vi "Example FPGA Main.vi"() -> ()   [LabVIEW 2010]
uses:
  <vilib>/Platform/TimedLoop/XDataNode/XDataNode.xnode
  <vilib>/Platform/TimedLoop/XDataNode/timing_clust.ctl
  <vilib>/Platform/TimedLoop/XDataNode/nitl_modes.ctl
  <vilib>/Platform/TimedLoop/XDataNode/wakeup.ctl
  <vilib>/Platform/TimedLoop/XDataNode/XDNodeRunTimeDep.lvlib
  <vilib>/NI Veristand/FPGA/NI_VS FPGA Support.lvlib
  <userlib>/_NI VeriStand FPGA Support/NI VeriStand FPGA Clock Support/NI_VS FPGA Clock Support.lvlib
panel:
  in  "PWM9 In Timeout":u32=40000
  out "PWM9 In DC Packet":u64
  out "PWM9 In Freq Packet":u64
  in  "PWM10 In Timeout":u32=40000
  out "PWM10 In DC Packet":u64
  out "PWM10 In Freq Packet":u64
  in  "PWM11 In Timeout":u32=40000
  out "PWM11 In DC Packet":u64
  out "PWM11 In Freq Packet":u64
  in  "PWM8 In Timeout":u32=40000
  out "PWM8 In DC Packet":u64
  out "PWM8 In Freq Packet":u64
  in  "PWM7 In Timeout":u32=40000
  out "PWM7 In DC Packet":u64
  out "PWM7 In Freq Packet":u64
  out "PWM6 In Freq Packet":u64
  in  "PWM6 In Timeout":u32=40000
  out "PWM6 In DC Packet":u64
  in  "Freq_Variable Freq Pkt":u64
  in  "DC Param DO5":u32
  in  "DC Param DO4":u32
  in  "Freq Param DO2":u32
  in  "Freq Param DO3":u32
  in  "DC_Variable DC Pkt":u64
  in  "Both_Variable DC Pkt":u64
  in  "Both_Variable Freq Pkt":u64
  in  "Generate IRQ":bool
  in  "Use External Timing":bool
  in  "Write to  RTSI":bool
  in  "Loop Rate (usec)":u32
  in  "Start":bool
  # "Pulse Generation"
  # "Pulse Generation"
  # "Configuration"
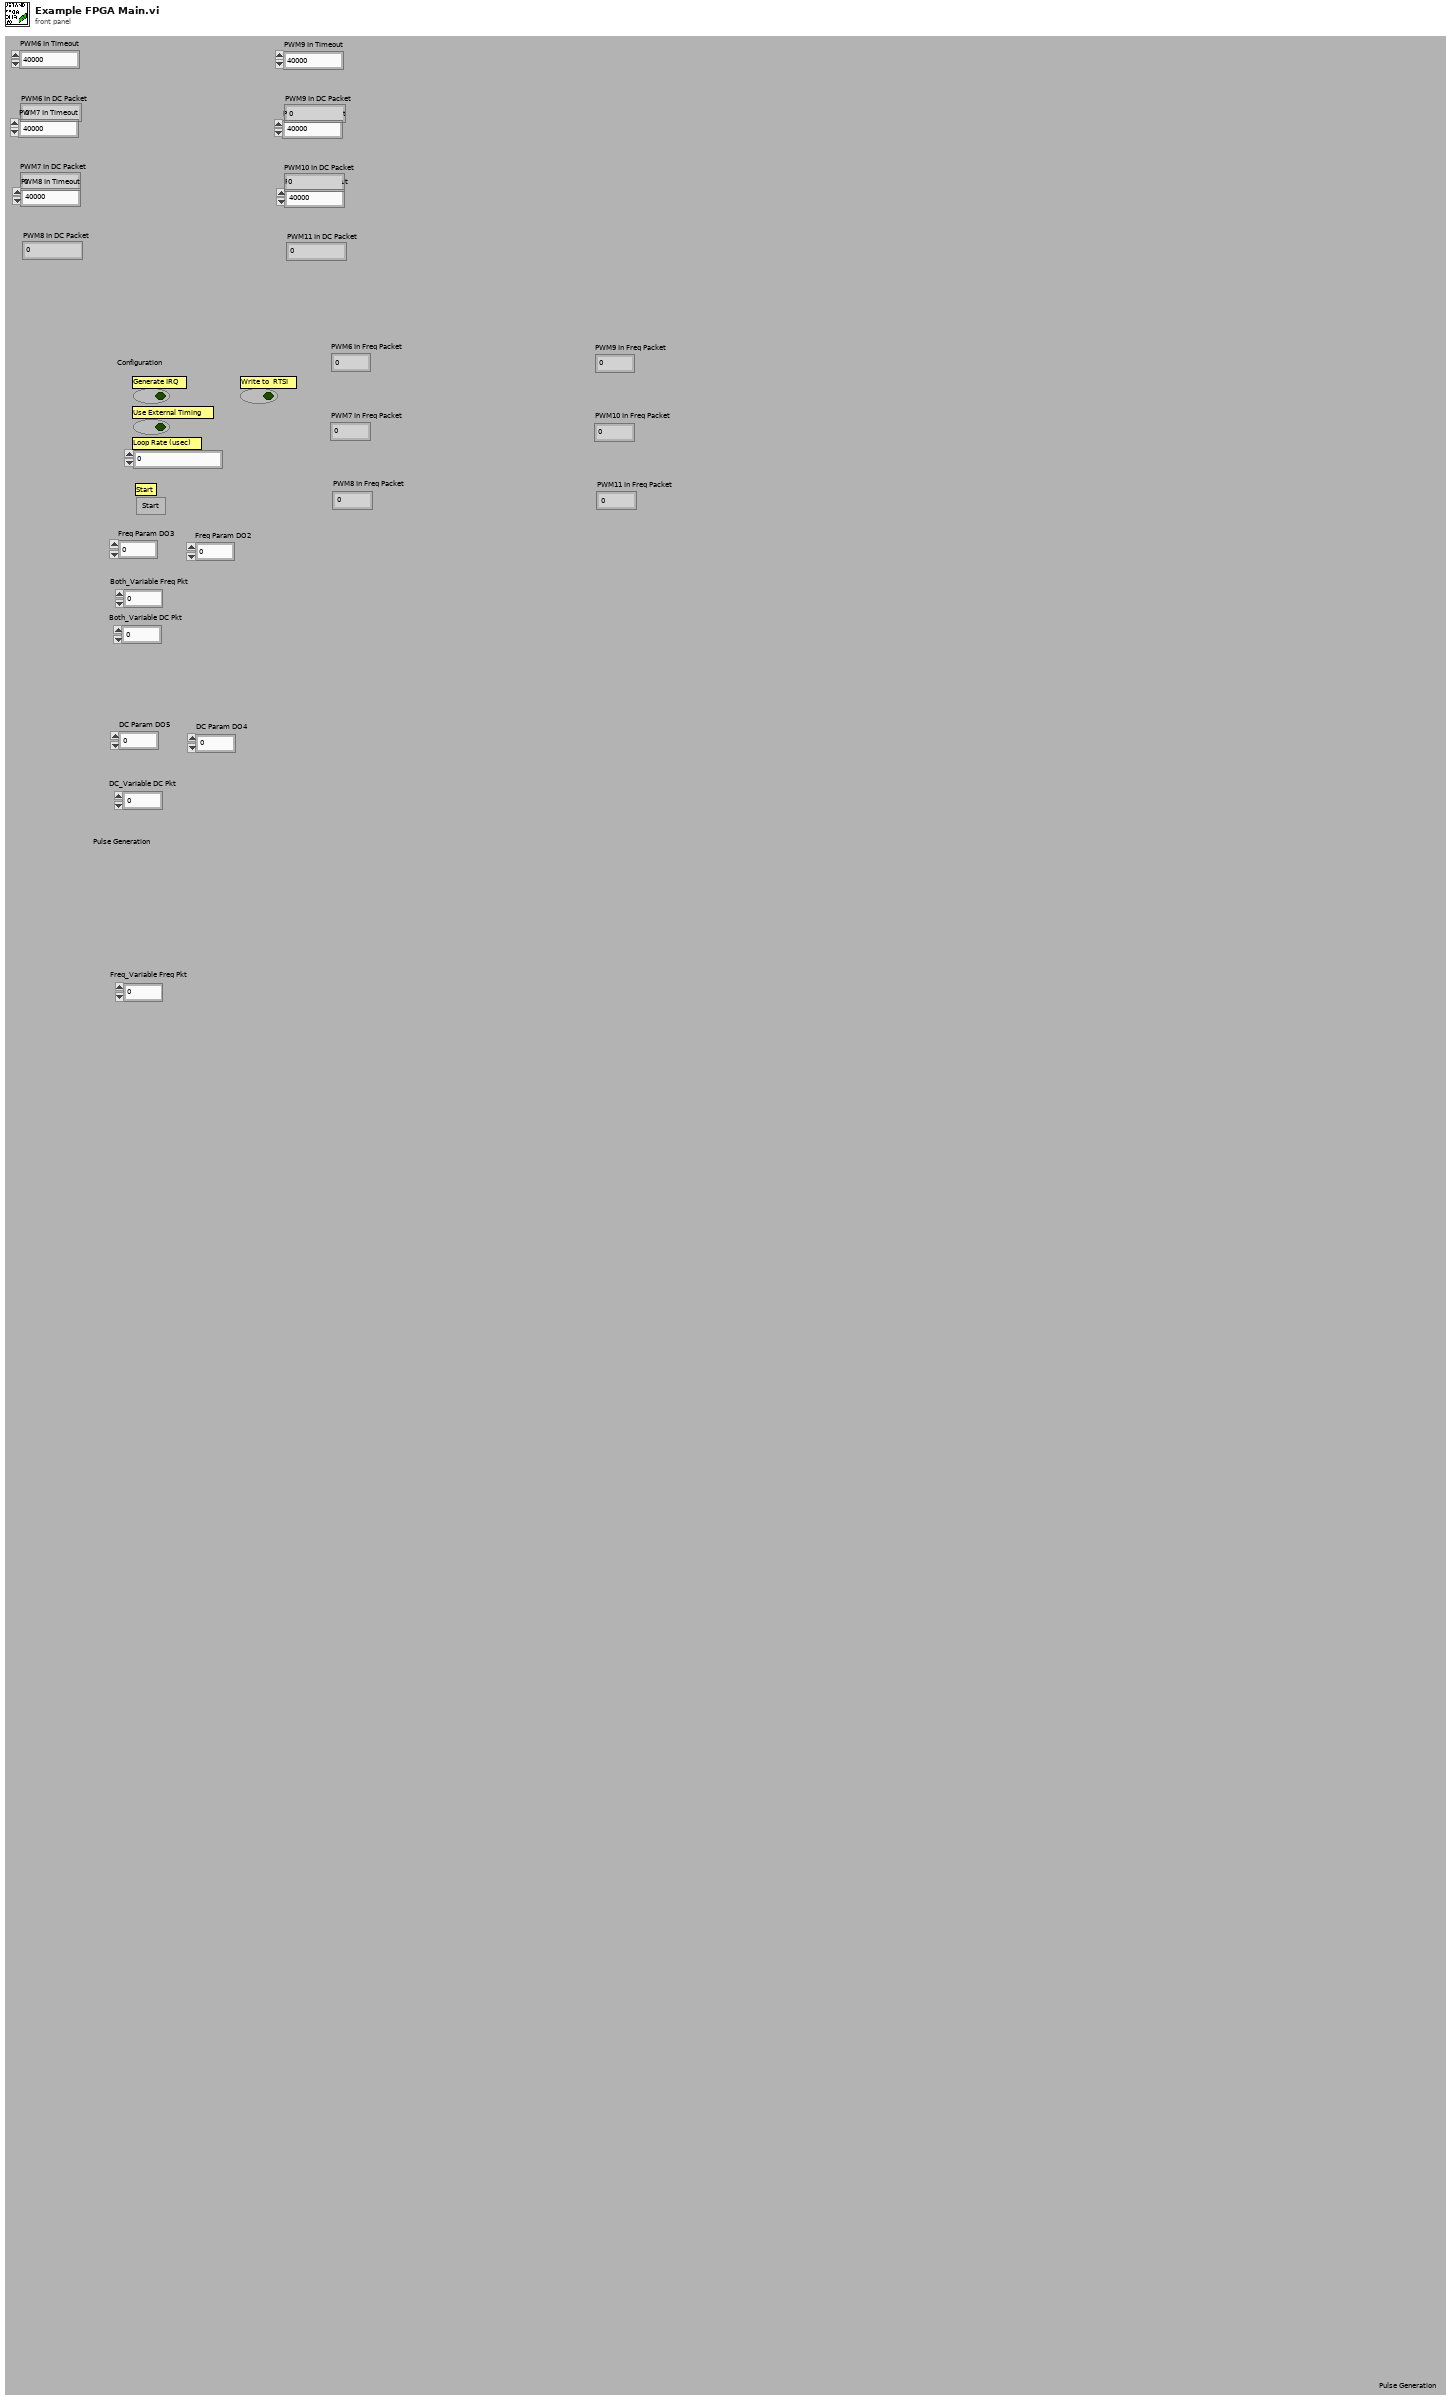
[diagram p1: front panel]
types:
  T1 = typedef "XDNodeRunTimeDep.lvlib/timing_clust.ctl" = cluster{"Expected End [f-1]":u64, "Actual End [f-1]":u64, "Finished Late? [f-1]":bool, "Expected End [i-1]":u64, "Actual End [i-1]":u64, "Finished Late? [i-1]":bool, "Expected Start [i]":u64, "Actual Start [i]":u64, "Expected Start [f]":u64, "Actual Start [f]":u64, "Source Name":string, "Structure Name":string, "Period":i64, "Deadline":i64, "Offset":i64, "Start":i64, "Priority":i32, "Timeout":i32, "Mode":T2, "Wakeup Reason":T3, "Error":errorcluster, "Source Type":string, "Secondary Source Type":string, "Global End Time":u64, "Global Start Time":u64, "Frame Duration":u64, "Iteration Duration":u64, "Assigned CPU":i32, "I/O Scan Engine Mode":u32}
  T2 = typedef "XDNodeRunTimeDep.lvlib/nitl_modes.ctl" = enum32{"No Change", "Process missed periods, maintain original phase", "Discard missed periods, maintain original phase", "Process missed periods, ignore original phase", "Discard missed periods, ignore original phase"}
  T3 = typedef "XDNodeRunTimeDep.lvlib/wakeup.ctl" = enum32{"Normal", "Aborted", "Asynchronous wakeup", "Timing source error", "Timed loop error", "Timeout"}
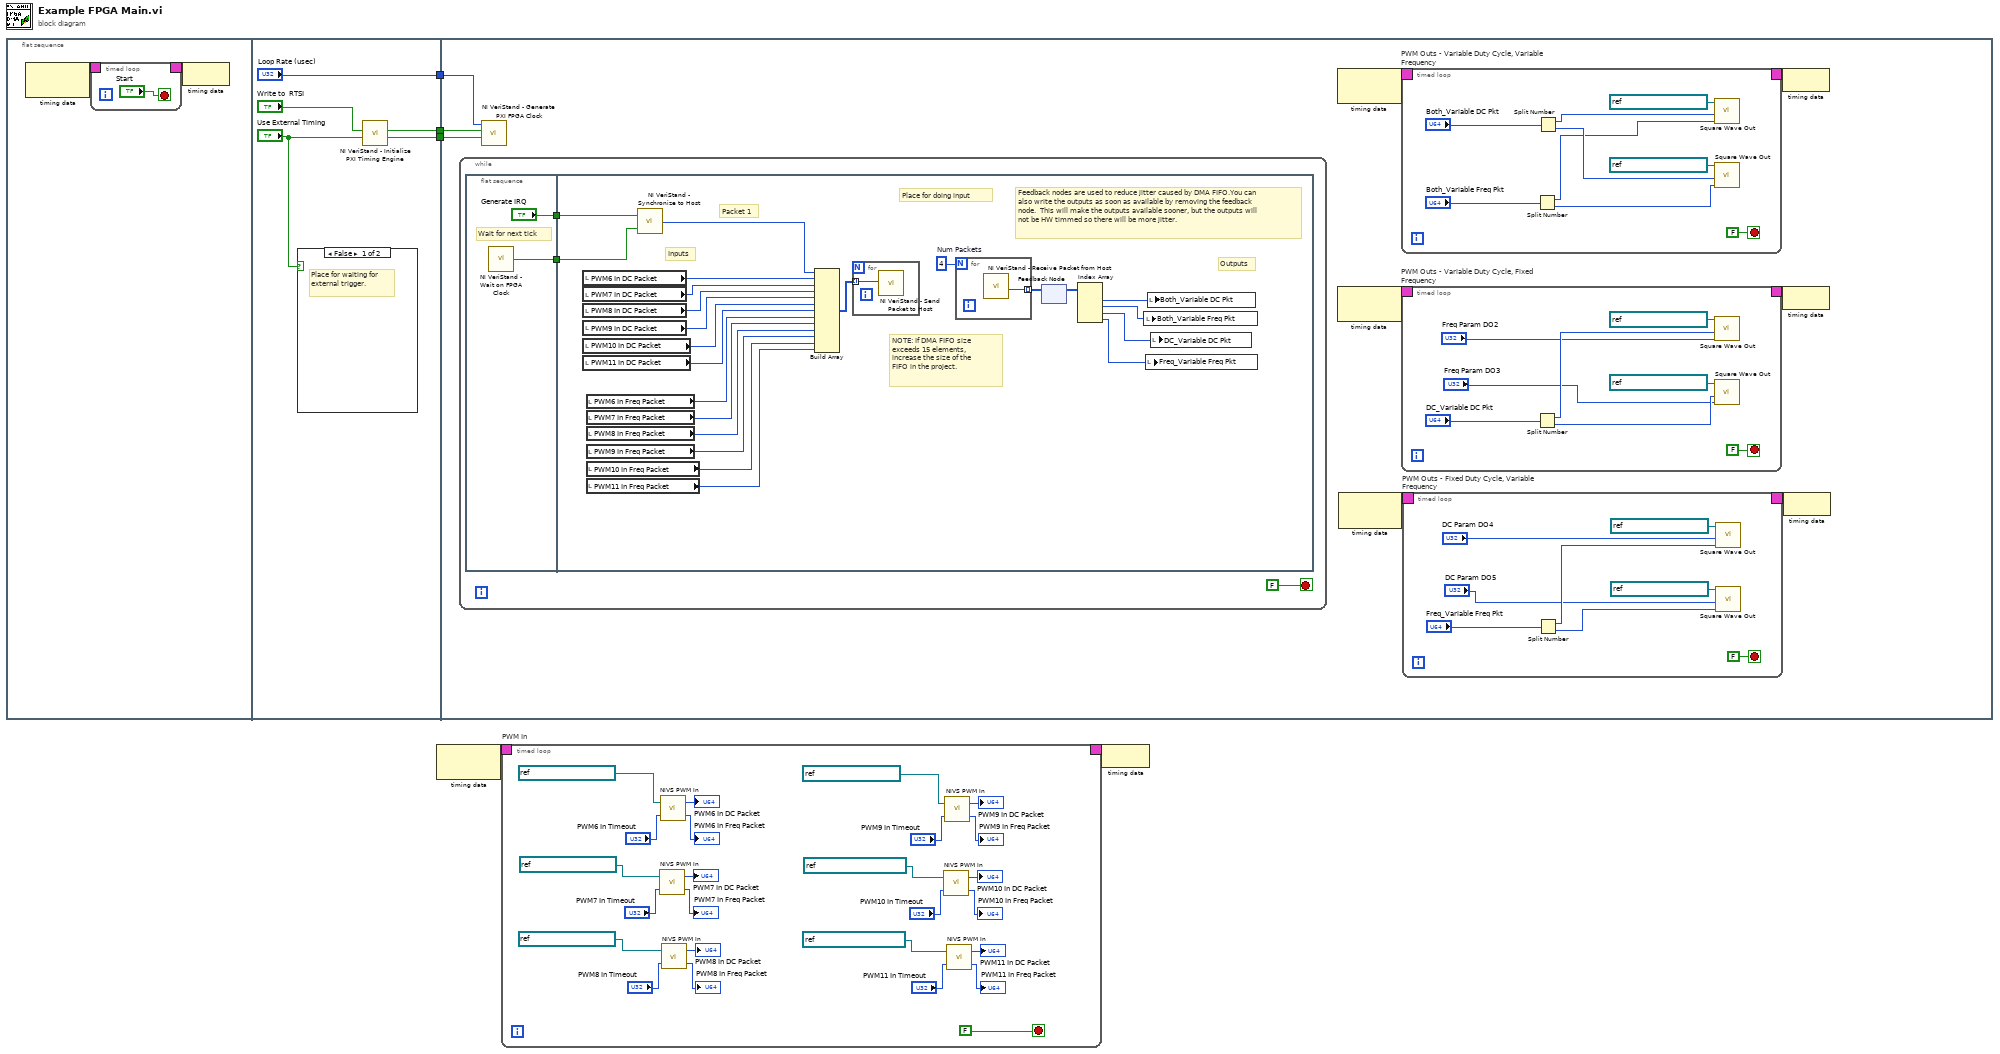
[diagram p0: block diagram]
diagram:
  n1 = flat-sequence {
    tunnel: [w14] -> w5
    tunnel: ["Loop Rate (usec)"] -> w4
    tunnel: [w13] -> w3
    tunnel: w5 -> [w26]
    tunnel: w4 -> [w25]
    tunnel: w3 -> [w24]
    frame #0 {
      n2 = node-c288() -> (w7:T1)  [unwired: 1 out]
      n3 = timed-loop {
        timing: w7 -> [_]
        timing-out: [_] -> w6
        stop <- "Start" stop-if-true
      }
      n4 = node-c288(w6) -> ()
    }
    frame #1 {
      n5 = case shown="False" "Use External Timing" {
        frame False {
          # "Place for waiting for external trigger."
        }
        frame True {
          # "Do not wait on trigger when externally timed."
        }
      }
      n6 = call <userlib>:"NI VeriStand - Initialize PXI Timing Engine.vi"("Use External Timing In"="Use External Timing", "Write to  RTSI In"="Write to  RTSI") -> ("Use External Timing Out"=w14:bool, "Write to  RTSI Out"=w13:bool)  [unwired: 8 in]
    }
    frame #2 {
      n7 = while {
        stop <- FALSE stop-if-true
        n8 = flat-sequence {
          tunnel: ["Generate IRQ"] -> w65
          tunnel: [w67] -> w64
          tunnel: w65 -> [w91]
          tunnel: w64 -> [w90]
          frame #0 {
            # "Wait for next tick"
            n9 = call <userlib>:"NI VeriStand - Wait on FPGA Clock.vi"() -> ("Clock Ticked"=w67:bool)
          }
          frame #1 {
            w89 = 4  # Num Packets
            # "Packet 1"
            # "Inputs"
            # "Outputs"
            # "NOTE: If DMA FIFO size exceeds 15 elements, increase the size of the FIFO in the project."
            # "Feedback nodes are used to reduce jitter caused by DMA FIFO.You can also write the outputs as soon as available by removing the feedback node.  This will make the outputs available sooner, but the outputs will not be HW timmed so there will be more jitter."
            # "Place for doing input"
            n10 = local read "PWM6 In DC Packet"() -> (w80:u64)
            n11 = local read "PWM7 In DC Packet"() -> (w79:u64)
            n12 = local read "PWM8 In DC Packet"() -> (w78:u64)
            n13 = local read "PWM9 In DC Packet"() -> (w77:u64)
            n14 = local read "PWM10 In DC Packet"() -> (w76:u64)
            n15 = local read "PWM11 In DC Packet"() -> (w75:u64)
            n16 = local read "PWM6 In Freq Packet"() -> (w74:u64)
            n17 = local read "PWM7 In Freq Packet"() -> (w73:u64)
            n18 = local read "PWM8 In Freq Packet"() -> (w72:u64)
            n19 = local read "PWM9 In Freq Packet"() -> (w71:u64)
            n20 = local read "PWM10 In Freq Packet"() -> (w70:u64)
            n21 = local read "PWM11 In Freq Packet"() -> (w69:u64)
            n22 = call <userlib>:"NI VeriStand - Synchronize to Host.vi"("Clock Ticked"=w90, "Generate IRQ"=w91) -> ("Is Late?"=w85:u64)
            n23 = Build Array(w85, w80, w79, w78, w77, w76, w75, w74, w73, w72, w71, w70, w69) -> (w88:u64[])
            n24 = for {
              tunnel: w88 -> [w92] mode=indexing
              n25 = call <vilib>:"NI VeriStand - Send Packet to Host.vi"("Element"=w92) -> ()  [unwired: 2 in, 9 out]
            }
            n26 = for {
              N: w89 -> [_]
              tunnel: [w93] -> w86 mode=indexing
              n27 = call <vilib>:"NI VeriStand - Receive Packet from Host.vi"() -> ("Element"=w93:u64)  [unwired: 2 in, 9 out]
            }
            n28 = feedback-in #1(w86) -> ()
            n29 = feedback #1() -> (w87:u64[])  [unwired: 1 in]
            n30 = Index Array(array=w87) -> (element #1=w84:u64, element #2=w83:u64, element #3=w82:u64, element #4=w81:u64)  [unwired: 4 in]
            n31 = local write "Both_Variable Freq Pkt"(w83) -> ()
            n32 = local write "Freq_Variable Freq Pkt"(w81) -> ()
            n33 = local write "Both_Variable DC Pkt"(w84) -> ()
            n34 = local write "DC_Variable DC Pkt"(w82) -> ()
          }
        }
      }
      n35 = call <userlib>:"NI VeriStand - Generate PXI FPGA Clock.vi"("Use External Timing"=w26, "Write to  RTSI"=w24, "Loop Rate (usec)"=w25) -> ()  [unwired: 9 in]
      n36 = node-c288() -> (w23:T1)  [unwired: 1 in]
      n37 = node-c288() -> (w21:T1)  [unwired: 1 in]
      n38 = node-c288() -> (w19:T1)  [unwired: 1 in]
      n39 = timed-loop "PWM Outs - Variable Duty Cycle, Variable Frequency" {
        timing: w23 -> [_]
        timing-out: [_] -> w22
        stop <- FALSE ("stop") stop-if-true
        n40 = Split Number(x="Both_Variable Freq Pkt") -> (hi(x)=w51:u32, lo(x)=w52:u32)
        n41 = Split Number(x="Both_Variable DC Pkt") -> (hi(x)=w54:u32, lo(x)=w53:u32)
        n42 = call "Square Wave Out.vi"("Frequency"=w51, "Duty Cycle"=w54, "FPGA I/O"=refnum<k21> "Connector1/DIO0") -> ()  [unwired: 9 in]
        n43 = call "Square Wave Out.vi"("Frequency"=w52, "Duty Cycle"=w53, "FPGA I/O"=refnum<k21> "Connector1/DIO1") -> ()  [unwired: 9 in]
      }
      n44 = timed-loop "PWM Outs - Variable Duty Cycle, Fixed Frequency" {
        timing: w21 -> [_]
        timing-out: [_] -> w20
        stop <- FALSE ("stop") stop-if-true
        n45 = Split Number(x="DC_Variable DC Pkt") -> (hi(x)=w42:u32, lo(x)=w41:u32)
        n46 = call "Square Wave Out.vi"("Frequency"="Freq Param DO2", "Duty Cycle"=w42, "FPGA I/O"=refnum<k21> "Connector1/DIO2") -> ()  [unwired: 9 in]
        n47 = call "Square Wave Out.vi"("Frequency"="Freq Param DO3", "Duty Cycle"=w41, "FPGA I/O"=refnum<k21> "Connector1/DIO3") -> ()  [unwired: 9 in]
      }
      n48 = timed-loop "PWM Outs - Fixed Duty Cycle, Variable Frequency" {
        timing: w19 -> [_]
        timing-out: [_] -> w18
        stop <- FALSE ("stop") stop-if-true
        n49 = Split Number(x="Freq_Variable Freq Pkt") -> (hi(x)=w29:u32, lo(x)=w30:u32)
        n50 = call "Square Wave Out.vi"("Frequency"=w29, "Duty Cycle"="DC Param DO4", "FPGA I/O"=refnum<k21> "Connector1/DIO4") -> ()  [unwired: 9 in]
        n51 = call "Square Wave Out.vi"("Frequency"=w30, "Duty Cycle"="DC Param DO5", "FPGA I/O"=refnum<k21> "Connector1/DIO5") -> ()  [unwired: 9 in]
      }
      n52 = node-c288(w22) -> ()
      n53 = node-c288(w20) -> ()
      n54 = node-c288(w18) -> ()
    }
  }
  n55 = node-c288() -> (w2:T1)  [unwired: 1 out]
  n56 = timed-loop "PWM In" {
    timing: w2 -> [_]
    timing-out: [_] -> w1
    stop <- FALSE stop-if-true
    n57 = call "NIVS PWM In.vi"("PWM In Timeout"="PWM7 In Timeout", "FPGA I/O"=refnum<k21> "Connector1/DIO7" ("FPGA I/O In")) -> ("PWM In Freq Packet"=→"PWM7 In Freq Packet":u64, "PWM In DC Packet"=→"PWM7 In DC Packet":u64)
    n58 = call "NIVS PWM In.vi"("PWM In Timeout"="PWM6 In Timeout", "FPGA I/O"=refnum<k21> "Connector1/DIO6" ("FPGA I/O In")) -> ("PWM In Freq Packet"=→"PWM6 In Freq Packet":u64, "PWM In DC Packet"=→"PWM6 In DC Packet":u64)
    n59 = call "NIVS PWM In.vi"("PWM In Timeout"="PWM8 In Timeout", "FPGA I/O"=refnum<k21> "Connector1/DIO8" ("FPGA I/O In")) -> ("PWM In Freq Packet"=→"PWM8 In Freq Packet":u64, "PWM In DC Packet"=→"PWM8 In DC Packet":u64)
    n60 = call "NIVS PWM In.vi"("PWM In Timeout"="PWM10 In Timeout", "FPGA I/O"=refnum<k21> "Connector1/DIO10" ("FPGA I/O In")) -> ("PWM In Freq Packet"=→"PWM10 In Freq Packet":u64, "PWM In DC Packet"=→"PWM10 In DC Packet":u64)
    n61 = call "NIVS PWM In.vi"("PWM In Timeout"="PWM9 In Timeout", "FPGA I/O"=refnum<k21> "Connector1/DIO9" ("FPGA I/O In")) -> ("PWM In Freq Packet"=→"PWM9 In Freq Packet":u64, "PWM In DC Packet"=→"PWM9 In DC Packet":u64)
    n62 = call "NIVS PWM In.vi"("PWM In Timeout"="PWM11 In Timeout", "FPGA I/O"=refnum<k21> "Connector1/DIO11" ("FPGA I/O In")) -> ("PWM In Freq Packet"=→"PWM11 In Freq Packet":u64, "PWM In DC Packet"=→"PWM11 In DC Packet":u64)
  }
  n63 = node-c288(w1) -> ()
